vi "Curtin_FixCommas.vi"(11 "String In":string) -> (3 "String In 2":string)   [LabVIEW 2022 SP3]
panel:
  out "offset past match":i32
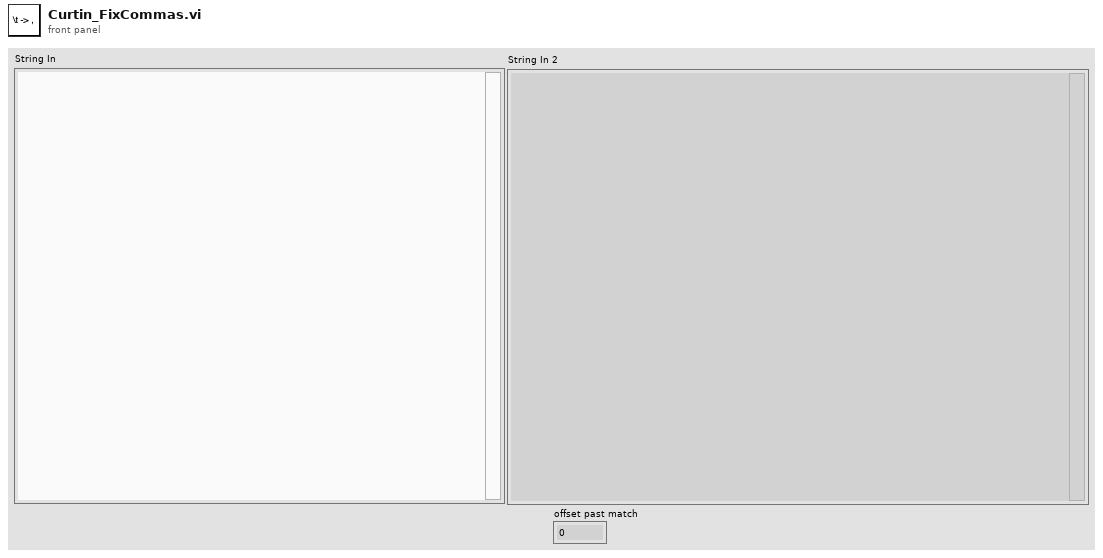
[diagram p1: front panel]
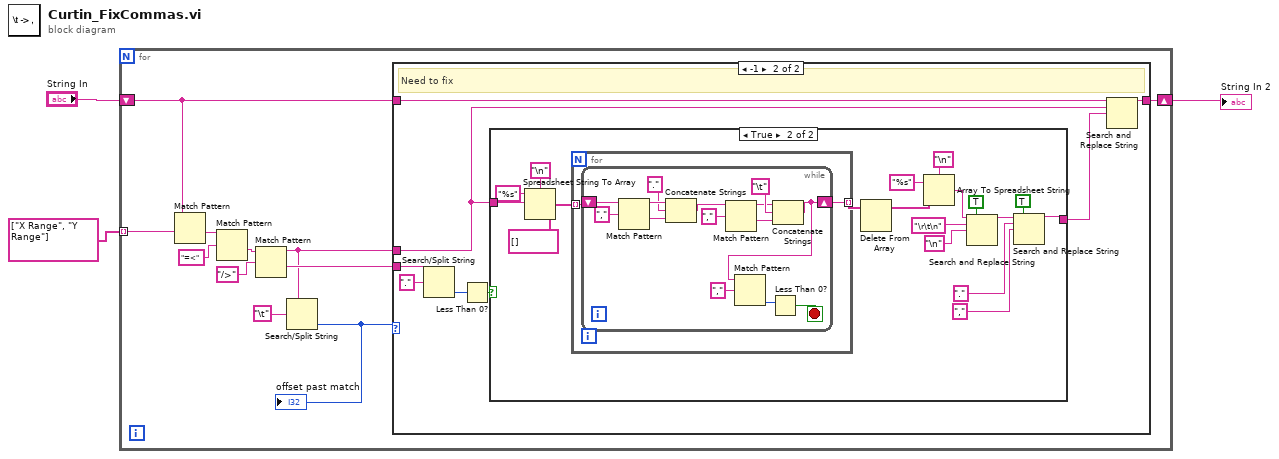
[diagram p0: block diagram]
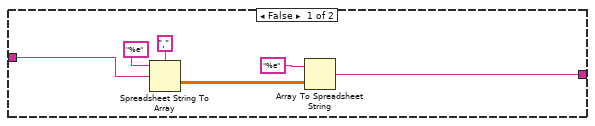
[diagram p3: hidden frame]
diagram:
  n1 = for {
    tunnel: string[] ["X Range", "Y Range"] -> [w10] mode=indexing
    shift-right: [w8] -> w2
    shift-left: "String In" -> [w9]
    n2 = Match Pattern(string=w9, regular expression=w10) -> (after substring=w11:string)  [unwired: 1 in, 3 out]
    n3 = Match Pattern(string=w11, regular expression="=<" ("format string")) -> (after substring=w12:string)  [unwired: 1 in, 3 out]
    n4 = Match Pattern(string=w12, regular expression="/>" ("format string")) -> (before substring=w4:string, after substring=w6:string)  [unwired: 1 in, 2 out]
    n5 = Search/Split String(string=w4, search string/char (-)="\t" ("format string")) -> (offset of match=w5:i32)  [unwired: 1 in, 2 out]
    "offset past match" <- w5
    n6 = case shown="-1" w5 {
      tunnel: w9 -> [w15 w20]
      tunnel: w6 -> [_ w19]
      tunnel: [w15 w17] -> w8
      tunnel: w4 -> [_ w16]
      frame 0, Default {
        # "All good"
      }
      frame -1 {
        # "Need to fix"
        n7 = Search/Split String(string=w19, search string/char (-)=".") -> (offset of match=w22:i32)  [unwired: 1 in, 2 out]
        n8 = Less Than 0?(x=w22) -> (x < 0?=w21:bool)
        n9 = case shown="True" w21 {
          tunnel: w16 -> [w28 w47]
          tunnel: [w24 w32] -> w18
          frame False {
            n10 = Spreadsheet String To Array(delimiter (Tab)=",", format string="%e", spreadsheet string=w28) -> (array=w25:dbl[][])  [unwired: 1 in]
            n11 = Array To Spreadsheet String(array=w25, 3:"%e" ("format string")) -> (spreadsheet string=w24:string)  [unwired: 1 in]
          }
          frame True {
            n12 = Spreadsheet String To Array(delimiter (Tab)="\n", format string="%s", spreadsheet string=w47, array type (2D Dbl)=string[] []) -> (array=w44:string[])
            n13 = for {
              tunnel: [w49] -> w36 mode=indexing
              tunnel: w44 -> [w48] mode=indexing
              n14 = while {
                shift-right: [w52] -> w49
                shift-left: w48 -> [w63]
                stop <- w50 stop-if-true
                n15 = Match Pattern(string=w63, regular expression=",") -> (before substring=w61:string, after substring=w60:string)  [unwired: 1 in, 2 out]
                n16 = Concatenate Strings(w61, "." ("string"), w60) -> (w54:string)
                n17 = Match Pattern(string=w54, regular expression=",") -> (before substring=w56:string, after substring=w57:string)  [unwired: 1 in, 2 out]
                n18 = Concatenate Strings(w56, "\t" ("string"), w57) -> (w52:string)
                n19 = Match Pattern(string=w52, regular expression=",") -> (offset past match=w51:i32)  [unwired: 1 in, 3 out]
                n20 = Less Than 0?(x=w51) -> (x < 0?=w50:bool)
              }
            }
            n21 = Delete From Array(array=w36) -> (array with subset deleted=w35:string[])  [unwired: 2 in, 1 out]
            n22 = Array To Spreadsheet String(delimiter (Tab)="\n", array=w35, 3:"%s" ("format string")) -> (spreadsheet string=w40:string)
            n23 = Search and Replace String(replace all?=TRUE ("replace all? (F)"), input string=w40, search string="\r\t\n" ("delimiter (Tab)"), replace string="\n" ("delimiter (Tab)")) -> (result string=w33:string)  [unwired: 4 in, 3 out]
            n24 = Search and Replace String(replace all?=TRUE ("replace all? (F)"), input string=w33, search string="." ("delimiter (Tab)"), replace string="," ("delimiter (Tab)")) -> (result string=w32:string)  [unwired: 4 in, 3 out]
          }
        }
        n25 = Search and Replace String(input string=w20, search string=w16, replace string=w18) -> (result string=w17:string)  [unwired: 5 in, 3 out]
      }
    }
  }
  "String In 2" <- w2
